vi "PendulumLoop.vi"() -> ()   [LabVIEW 2017, in "PendulumLoop.lvlib"]
uses:
  PendulumLoop.lvlib
  PendulomLoop.Data.ctl
  Render Model.PendulumData.ctl
  PendulumLoop.Outputs.ci.vi
  Communication/Communication.lvlib
panel:
  out "3D Picture":refnum<vi>(3d-picture)
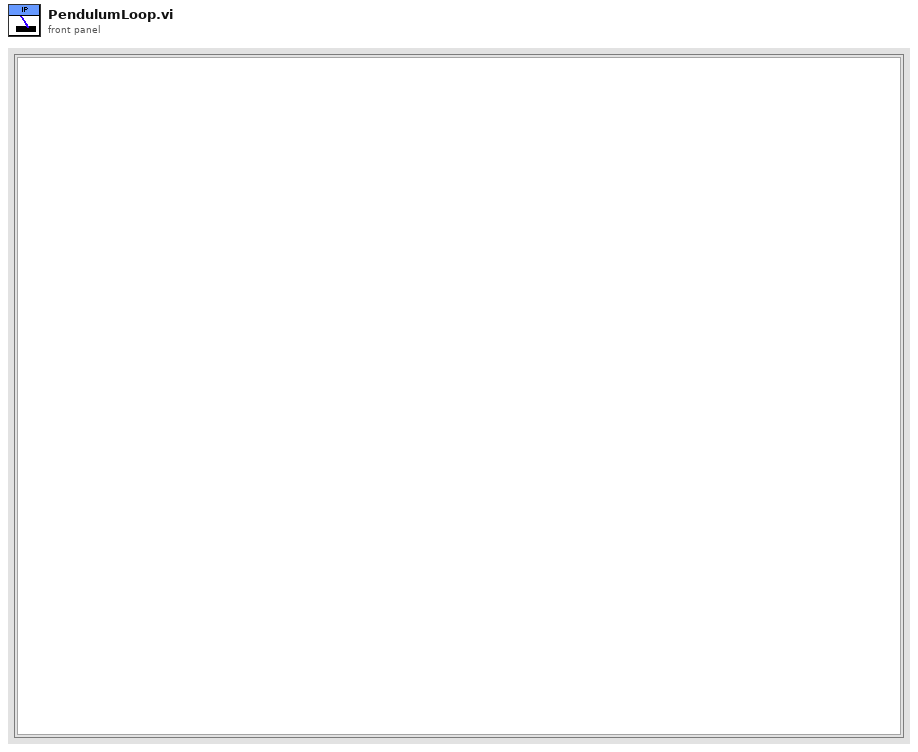
[diagram p1: front panel]
types:
  T1 = typedef "PendulumLoop.lvlib/PendulomLoop.Data.ctl" = cluster{"Initialized?":bool, "Pendulum Data":T2, "DLL Path":path, "plenght":dbl, "Cart X":dbl, "Reset Camera Flag":bool, "Cart Force":dbl}
  T2 = typedef "PendulumLoop.lvlib/Render Model.PendulumData.ctl" = cluster{"Angle":sgl, "Lenght":sgl, "X":sgl, "Y":sgl}
  T3 = cluster{"plenght":dbl, "cartMass":dbl, "pendulumMass":dbl, "angle":dbl}
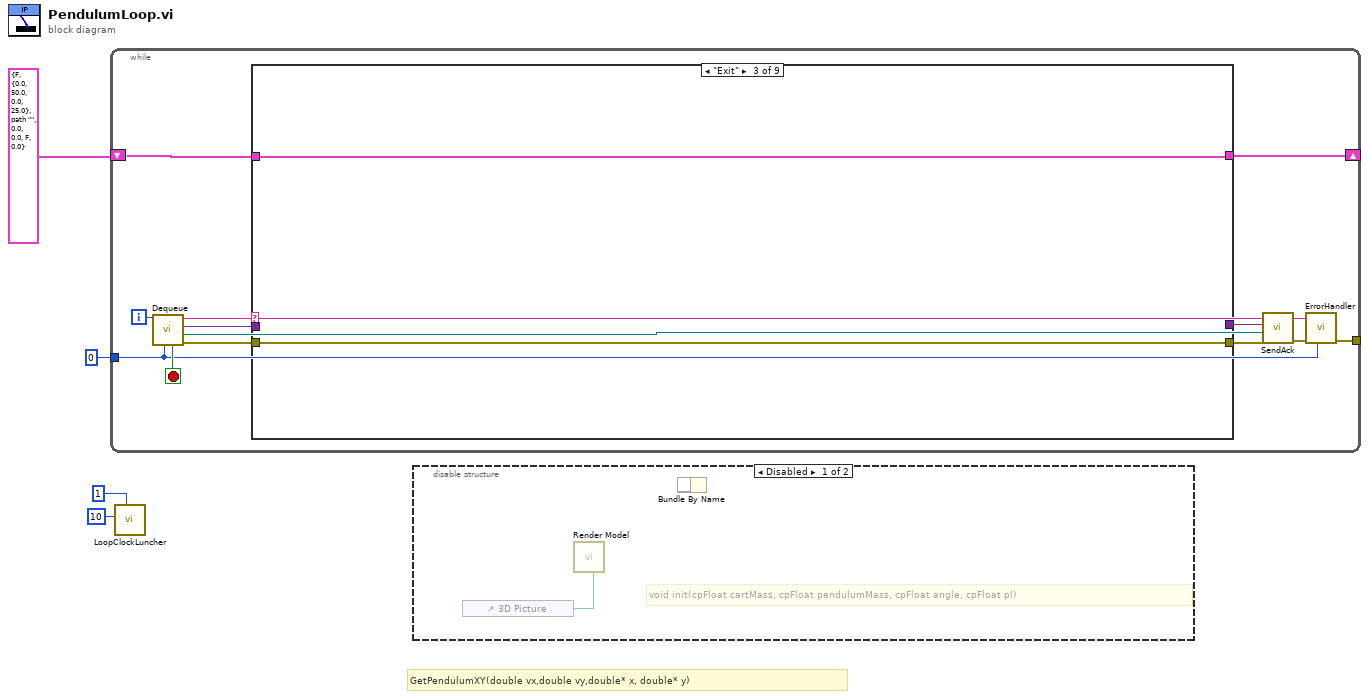
[diagram p0: block diagram]
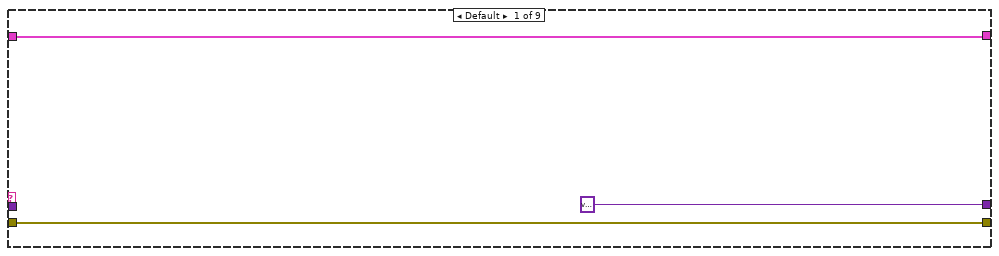
[diagram p3: hidden frame]
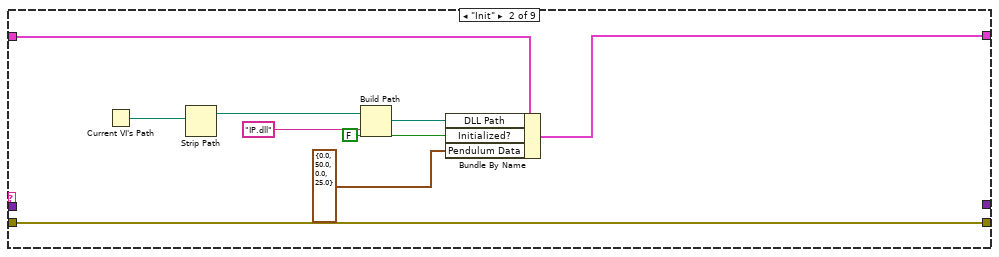
[diagram p4: hidden frame]
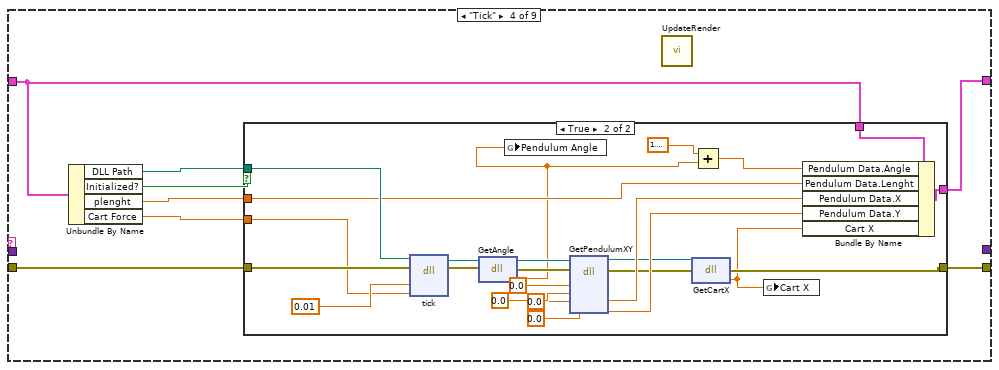
[diagram p5: hidden frame]
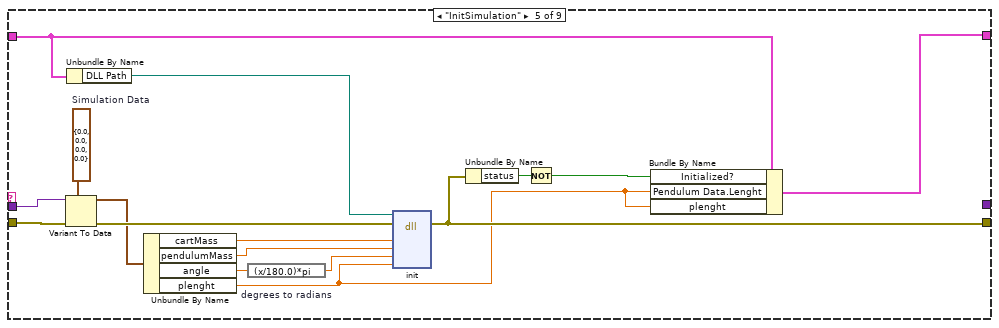
[diagram p7: hidden frame]
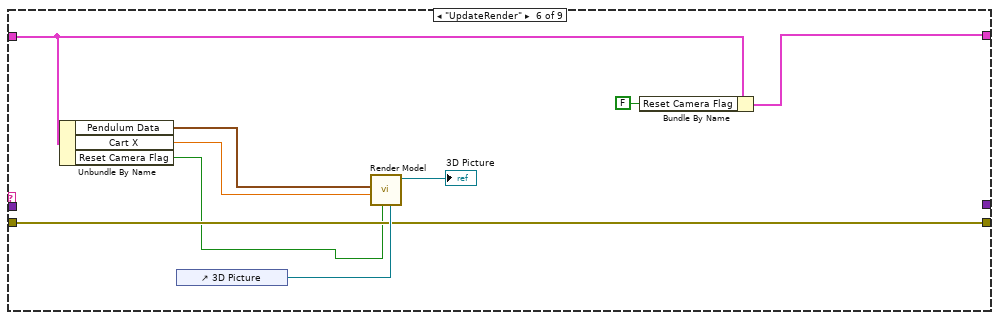
[diagram p8: hidden frame]
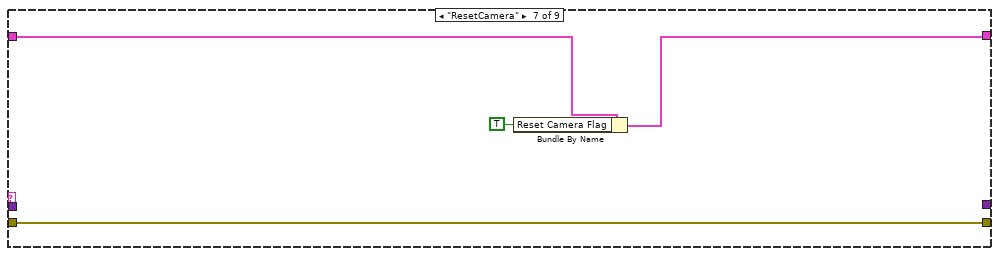
[diagram p9: hidden frame]
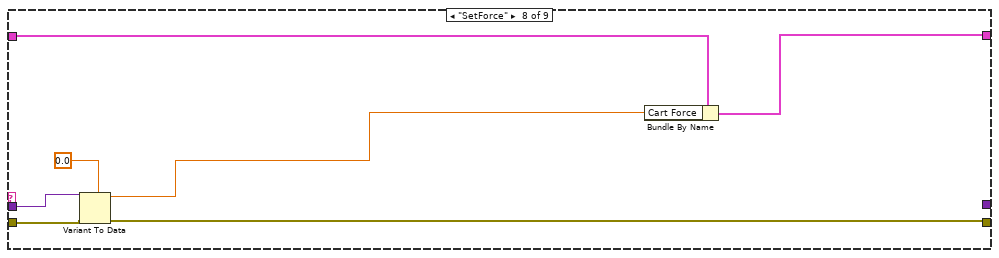
[diagram p10: hidden frame]
diagram:
  # "GetPendulumXY(double vx,double vy,double* x, double* y)"
  n1 = while {
    tunnel: 0 -> [w9]
    tunnel: [w11] -> _
    shift-right: [w6] -> _
    shift-left: T1 {"Initialized?"=FALSE, "Pendulum Data"={"Angle"=0.0, "Lenght"=50.0, "X"=0.0, "Y"=25.0}, "DLL Path"=path "", "plenght"=0.0, "Cart X"=0.0, "Reset Camera Flag"=FALSE, "Cart Force"=0.0} -> [w5]
    i -> [w10]
    stop <- w17 stop-if-true
    n2 = call "Dequeue.vi"("Instance"=w9, "Loop Counter"=w10) -> ("error out"=w14:errorcluster, "ResponseNotifcation"=w15:refnum<notifier>, "Data"=w16:variant, "Msg"=w8:string, "Exit?"=w17:bool)  [unwired: 5 in]
    n3 = case shown="\"Exit\"" w8 {
      tunnel: w16 -> [_ _ _ _ w74 _ _ w98 _]
      tunnel: w14 -> [w20 w29 w31 w37 w80 w86 w91 w99 w103]
      tunnel: [variant _ _ _ _ _ _ _ _] -> w13
      tunnel: [w20 w29 w31 w36 w72 w86 w91 w95 w103] -> w7
      tunnel: w5 -> [w18 w25 w30 w35 w73 w84 w94 w101 w102]
      tunnel: [w18 w21 w30 w33 w70 w82 w93 w100 w102] -> w6
      frame Default {
      }
      frame "Init" {
        n4 = Current VI's Path() -> (path=w28:path)
        n5 = Strip Path(path=w28) -> (stripped path=w27:path)  [unwired: 1 out]
        n6 = Build Path(base path=w27, name or relative path="IP.dll") -> (appended path=w24:path)
        n7 = Bundle By Name(cluster=w25, "DLL Path"=w24, "Initialized?"=FALSE, "Pendulum Data"=T2 {"Angle"=0.0, "Lenght"=50.0, "X"=0.0, "Y"=25.0}) -> (w21:T1)
      }
      frame "Exit" {
      }
      frame "Tick" {
        n8 = Unbundle By Name(w35) -> ("DLL Path"=w38:path, "Initialized?"=w39:bool, "plenght"=w34:dbl, "Cart Force"=w32:dbl)
        n9 = case shown="True" w39 {
          tunnel: w38 -> [_ w64]
          tunnel: w37 -> [w41 w63]
          tunnel: [w41 w47] -> w36
          tunnel: w35 -> [w40 w55]
          tunnel: w34 -> [_ w54]
          tunnel: [w40 w51] -> w33
          tunnel: w32 -> [_ w44]
          frame False {
          }
          frame True {
            n10 = dll-call lib="C:/Users/bartl/Desktop/Power 13-15/InvertedPendulum/PendulumLoop/IP.dll" fn="tick"(path in=w64, error in=w63, "dt"=0.01, "cartForce"=w44) -> (path out=w61:path, error out=w62:errorcluster)  [unwired: 4 in]
            n11 = dll-call lib="C:/Users/bartl/Desktop/Power 13-15/InvertedPendulum/PendulumLoop/IP.dll" fn="GetAngle"(path in=w61, error in=w62) -> (path out=w60:path, error out=w50:errorcluster, "return type"=w42:sgl)  [unwired: 1 in]
            n12 = global write "PendulumLoop.Outputs.ci.vi" "Pendulum Angle"(w42) -> ()
            n13 = dll-call lib="C:/Users/bartl/Desktop/Power 13-15/InvertedPendulum/PendulumLoop/IP.dll" fn="GetPendulumXY"(path in=w60, error in=w50, "vx"=0.0, "vy"=0.0, "x"=0.0, "y"=0.0) -> (path out=w49:path, error out=w48:errorcluster, "x"=w53:dbl, "y"=w52:dbl)  [unwired: 4 in]
            n14 = dll-call lib="C:/Users/bartl/Desktop/Power 13-15/InvertedPendulum/PendulumLoop/IP.dll" fn="GetCartX"(path in=w49, error in=w48) -> (error out=w47:errorcluster, "return type"=w43:sgl)  [unwired: 1 in, 1 out]
            n15 = Add(x=1.5707963267948966, y=w42) -> (x+y=w46:dbl)
            n16 = global write "PendulumLoop.Outputs.ci.vi" "Cart X"(w43) -> ()
            n17 = Bundle By Name(cluster=w55, "Pendulum Data.Angle"=w46, "Pendulum Data.Lenght"=w54, "Pendulum Data.X"=w53, "Pendulum Data.Y"=w52, "Cart X"=w43) -> (w51:T1)
          }
        }
        n18 = call "UpdateRender.vi"() -> ()  [unwired: 11 in, 1 out]
      }
      frame "InitSimulation" {
        w79 = T3 {"plenght"=0.0, "cartMass"=0.0, "pendulumMass"=0.0, "angle"=0.0}  # Simulation Data
        n19 = Variant To Data(error in=w80, type=w79, Variant=w74) -> (data=w77:T3, error out=w78:errorcluster)
        n20 = Unbundle By Name(w73) -> ("DLL Path"=w81:path)
        n21 = Unbundle By Name(w77) -> ("cartMass"=w76:dbl, "pendulumMass"=w75:dbl, "angle"=w69:dbl, "plenght"=w67:dbl)
        n22 = expression code="(x/180.0)*pi" "degrees to radians"(w69) -> (w66:dbl)
        n23 = dll-call lib="C:/Users/bartl/Desktop/Power 13-15/InvertedPendulum/PendulumLoop/IP.dll" fn="init"(path in=w81, error in=w78, "cartMass"=w76, "pendulumMass"=w75, "angle"=w66, "plenght"=w67) -> (error out=w72:errorcluster)  [unwired: 6 in, 1 out]
        n24 = Unbundle By Name(w72) -> ("status"=w71:bool)
        n25 = Not(x=w71) -> (.not. x?=w68:bool)
        n26 = Bundle By Name(cluster=w73, "Initialized?"=w68, "Pendulum Data.Lenght"=w67, "plenght"=w67) -> (w70:T1)
      }
      frame "UpdateRender" {
        n27 = Unbundle By Name(w84) -> ("Pendulum Data"=w88:T2, "Cart X"=w87:dbl, "Reset Camera Flag"=w85:bool)
        n28 = control-ref of="3D Picture"() -> (w90:refnum<vi>)
        n29 = call "Render Model.vi"("3D Picture 2"=w90, "Reset Camera"=w85, "Cart X"=w87, 10:w88) -> ("Scene Object Out"=→"3D Picture":refnum<vi>)  [unwired: 7 in]
        n30 = Bundle By Name(cluster=w84, "Reset Camera Flag"=FALSE) -> (w82:T1)
      }
      frame "ResetCamera" {
        n31 = Bundle By Name(cluster=w94, "Reset Camera Flag"=TRUE) -> (w93:T1)
      }
      frame "SetForce" {
        n32 = Variant To Data(error in=w99, type=0.0 ("Cart Force"), Variant=w98) -> (data=w96:dbl, error out=w95:errorcluster)
        n33 = Bundle By Name(cluster=w101, "Cart Force"=w96) -> (w100:T1)
      }
      frame "Error" {
      }
    }
    n34 = call "SendAck.vi"("error in (no error)"=w7, "Ack"=w15, "Variant"=w13) -> ("error out"=w12:errorcluster)  [unwired: 8 in]
    n35 = call "ErrorHandler.vi"("Instance"=w9, "error in (no error)"=w12, "Msg"=w8) -> ("error out"=w11:errorcluster)  [unwired: 8 in]
  }
  n36 = call "LoopClockLuncher.vi"("Loop VI Depth"=1, "milliseconds to wait"=10) -> ()  [unwired: 8 in, 2 out]
  n37 = disable-structure shown="Disabled" {
    frame Disabled {
      # "void init(cpFloat cartMass, cpFloat pendulumMass, cpFloat angle, cpFloat pl)"
      n38 = control-ref of="3D Picture"() -> (w104:refnum<vi>)
      n39 = call "Render Model.vi"("3D Picture 2"=w104) -> ()  [unwired: 10 in, 1 out]
      n40 = Bundle By Name() -> ()  [unwired: 2 in, 1 out]
    }
    frame Enabled {
    }
  }
